vi "Start Batch Car Wash.vi"(8 "error in (no error)":errorcluster, 10 "String":string, 11 "Car Wash Model in":refnum<class "Car Wash Model.lvclass">) -> (0 "error out":errorcluster, 3 "Car Wash Model out":refnum<class "Car Wash Model.lvclass">)   [LabVIEW 2019, in "Car Wash Model.lvclass"]
uses:
  <vilib>/gpm_packages/@cs/Car-wash/Source/Car Wash Model/Car Wash Model/Car Wash Model.lvclass
  C:/Program Files/National Instruments/LabVIEW 2019/vi.lib/gpm_packages/@cs/mva-core/Source/IModel/IModel/IModel.lvclass
  <vilib>/gpm_packages/@cs/Car-wash/Source/Car Wash Model/Car Wash Model/Car Wash Model.lvclass/Car Wash Model.ctl
  <vilib>/gpm_packages/@cs/Car-wash/Source/iProcess Model/iProcess Model Messages/Create Process from File Msg/Create Process from File Msg.lvclass/Create Process from File Msg.ctl
  <vilib>/ActorFramework/Message Enqueuer/Message Enqueuer.lvclass/Message Enqueuer.ctl
  <vilib>/gpm_packages/@cs/mva-core/Source/IMediator/ISubscriptionPolicy/ISubscriptionPolicy.lvclass/ISubscriptionPolicy.ctl
  <vilib>/gpm_packages/@cs/mva-core/Source/IObserver/IObserver/IObserver.lvclass/IObserver.ctl
  <vilib>/gpm_packages/@cs/mva-core/Source/IModel/IModel/IModel.lvclass/IModel.ctl
  <vilib>/gpm_packages/@cs/mva-core/Source/IMediator/PublishRequest/PublishRequest.lvclass/PublishRequest.ctl
  <vilib>/gpm_packages/@cs/mva-core/Source/IMediator/IMediator Messages/Publish Msg/Publish Msg.lvclass/Publish Msg.ctl
  <vilib>/gpm_packages/@cs/actor-framework-messages/Source/RoundTripMessage/RoundTripMessage.lvclass/RoundTripMessage.ctl
  <vilib>/ActorFramework/Message Enqueuer/Enqueue.vi
  <vilib>/gpm_packages/@cs/mva-core/Source/IMediator/IMediator Messages/Publish Msg/Send Pre-Addressed Publish.vi
  <vilib>/gpm_packages/@cs/mva-core/Source/IObserver/IObserver/Read Unique ID.vi
  <vilib>/gpm_packages/@cs/mva-core/Source/IMediator/PublishRequest/Pack Publish Request.vi
  <vilib>/gpm_packages/@cs/actor-framework-messages/Source/RoundTripMessage/Return Round-Trip Message.vi
  <vilib>/gpm_packages/@cs/Car-wash/Source/iProcess Model/iProcess Model/iProcess Model.lvclass
  <vilib>/gpm_packages/@cs/Car-wash/Source/iProcess Model/iProcess Model Messages/Create Process from File Msg/Create Process from File Msg.lvclass
  C:/Program Files/National Instruments/LabVIEW 2019/vi.lib/ActorFramework/Message/Message.lvclass
  <vilib>/gpm_packages/@cs/Car-wash/Source/iProcess Model/iProcess Model Messages/Start Process Msg/Start Process Msg.lvclass
  <vilib>/gpm_packages/@cs/mva-core/Source/IModel/IModel/IModel.lvclass
  C:/Program Files/National Instruments/LabVIEW 2019/vi.lib/gpm_packages/@cs/mva-core/Source/IObserver/IObserver/IObserver.lvclass
  <vilib>/gpm_packages/@cs/mva-core/Source/IMediator/IMediator Messages/Publish Msg/Publish Msg.lvclass
  C:/Program Files/National Instruments/LabVIEW 2019/vi.lib/gpm_packages/@cs/actor-framework-messages/Source/RoundTripMessage/RoundTripMessage.lvclass
  <vilib>/gpm_packages/@cs/actor-framework-messages/Source/RoundTripMessage/RoundTripMessage.lvclass
  <vilib>/ActorFramework/Message Priority Queue/Priority Enqueue.vi
  <vilib>/Utility/error.llb/Error Cluster From Error Code.vi
  <vilib>/gpm_packages/@cs/mva-core/Source/IMediator/PublishRequest/PublishRequest.lvclass
  <vilib>/gpm_packages/@cs/mva-core/Source/IMediator/ISubscriptionPolicy/ISubscriptionPolicy.lvclass
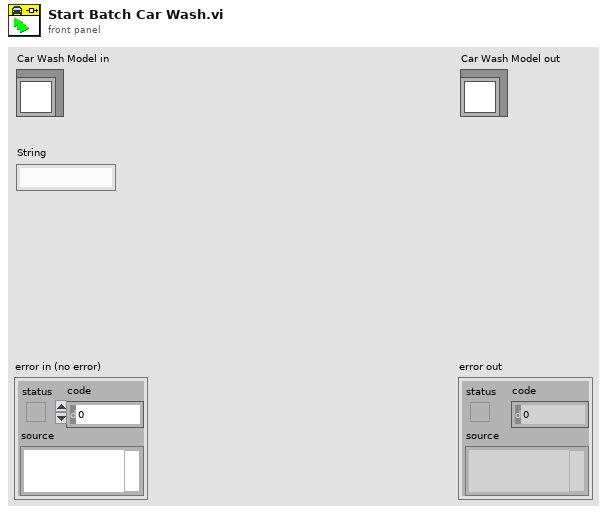
[diagram p1: front panel]
types:
  T1 = typedef "IMediator.lvlib/ISubscriptionPolicy.lvclass/ISubscriptionPolicy Reference.ctl" = refnum<data-value>
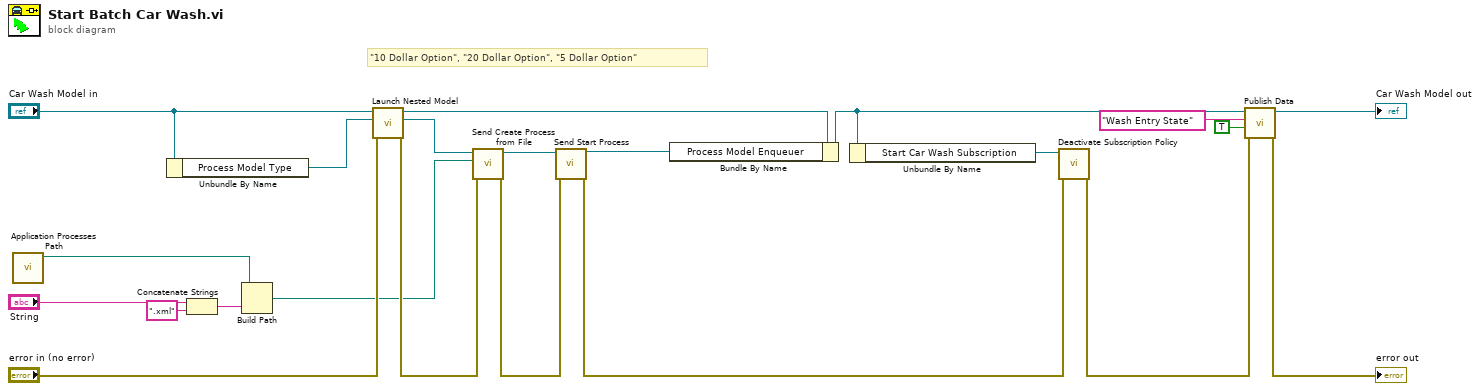
[diagram p0: block diagram]
diagram:
  # "\"10 Dollar Option\", \"20 Dollar Option\", \"5 Dollar Option\""
  n1 = call <vilib>:"Application Processes Path.vi"() -> ("Application Processes Path"=w3:path)  [unwired: 11 in]
  n2 = Unbundle By Name("Car Wash Model in") -> ("Process Model Type"=w21:refnum<class "iProcess Model.lvclass">)
  n3 = Concatenate Strings("String", ".xml" ("string")) -> (w2:string)
  n4 = Build Path(base path=w3, name or relative path=w2) -> (appended path=w1:path)
  n5 = call-dynamic "Launch Nested Model.vi"("error in (no error)"="error in (no error)", "Model to Launch"=w21, "IModel in"="Car Wash Model in") -> ("error out"=w8:errorcluster, "Nested Model Enqueuer"=w19:refnum<class "Message Enqueuer.lvclass">, "IModel out"=w12:refnum<class "Car Wash Model.lvclass">)  [unwired: 6 in]
  n6 = call <vilib>:"Send Create Process from File.vi"("error in (no error)"=w8, "Process"=w1, "Message Enqueuer"=w19) -> ("error out"=w7:errorcluster, "Message Enqueuer out"=w18:refnum<class "Message Enqueuer.lvclass">)  [unwired: 7 in]
  n7 = call <vilib>:"Send Start Process.vi"("error in (no error)"=w7, "Message Enqueuer"=w18) -> ("error out"=w6:errorcluster, "Message Enqueuer out"=w9:refnum<class "Message Enqueuer.lvclass">)  [unwired: 8 in]
  n8 = Bundle By Name(cluster=w12, "Process Model Enqueuer"=w9) -> (w16:refnum<class "Car Wash Model.lvclass">)
  n9 = Unbundle By Name(w16) -> ("Start Car Wash Subscription"=w17:T1)
  n10 = call <vilib>:"Deactivate Subscription Policy.vi"("error in (no error)"=w6, "Subscription Policy"=w17) -> ("error out"=w15:errorcluster)  [unwired: 9 in]
  n11 = call <vilib>:"Publish Data.vi"("error in (no error)"=w15, "Data to Publish"=TRUE, "Datum Name"="Wash Entry State" ("Datum Name (\"\"=Use Control Label)"), "IModel in"=w16) -> ("error out"=→"error out":errorcluster, "IModel out"=→"Car Wash Model out":refnum<class "Car Wash Model.lvclass">)  [unwired: 6 in]
